vi "Prebuild Action VI.vi"(6 "Top Level/Always Included VIs":path[](array[path]), 7 "Main Destination Path":path, 9 "Target Name":string, 10 "Build Specification Name":string, 11 "Project Path":path) -> (0 "error out":errorcluster)   [LabVIEW 2018]
uses:
  <vilib>/AppBuilder/AB_API_Simple/Build Specification Version.ctl
  <vilib>/AppBuilder/AB_API_Simple/Get Build Specification Version (project reference).vi
  <vilib>/AppBuilder/AB_API_Simple/Set Build Specification Version (project reference).vi
  <vilib>/AppBuilder/AB_API_Simple/NI_App_Builder_API.lvlib
  <vilib>/Utility/config.llb/NI_LVConfig.lvlib
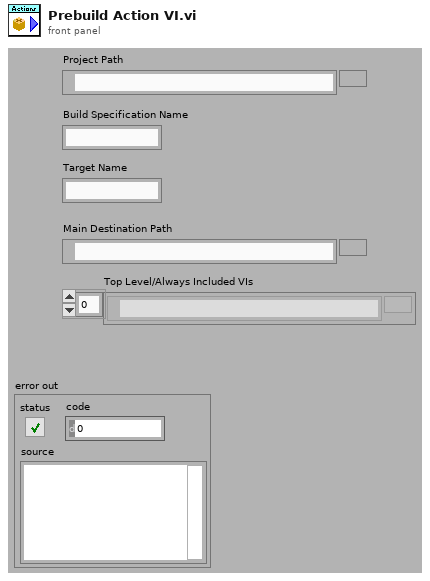
[diagram p1: front panel]
types:
  T1 = typedef "NI_App_Builder_API.lvlib/Build Specification Version.ctl" = cluster{"Major":u16, "Minor":u16, "Fix":u16, "Build":u16}
  T2 = cluster{"Major":bool, "Minor":bool, "Fix":bool, "Build":bool}
  T3 = typedef "NI_LVConfig.lvlib/Config Data RefNum.ctl" = refnum<k1>
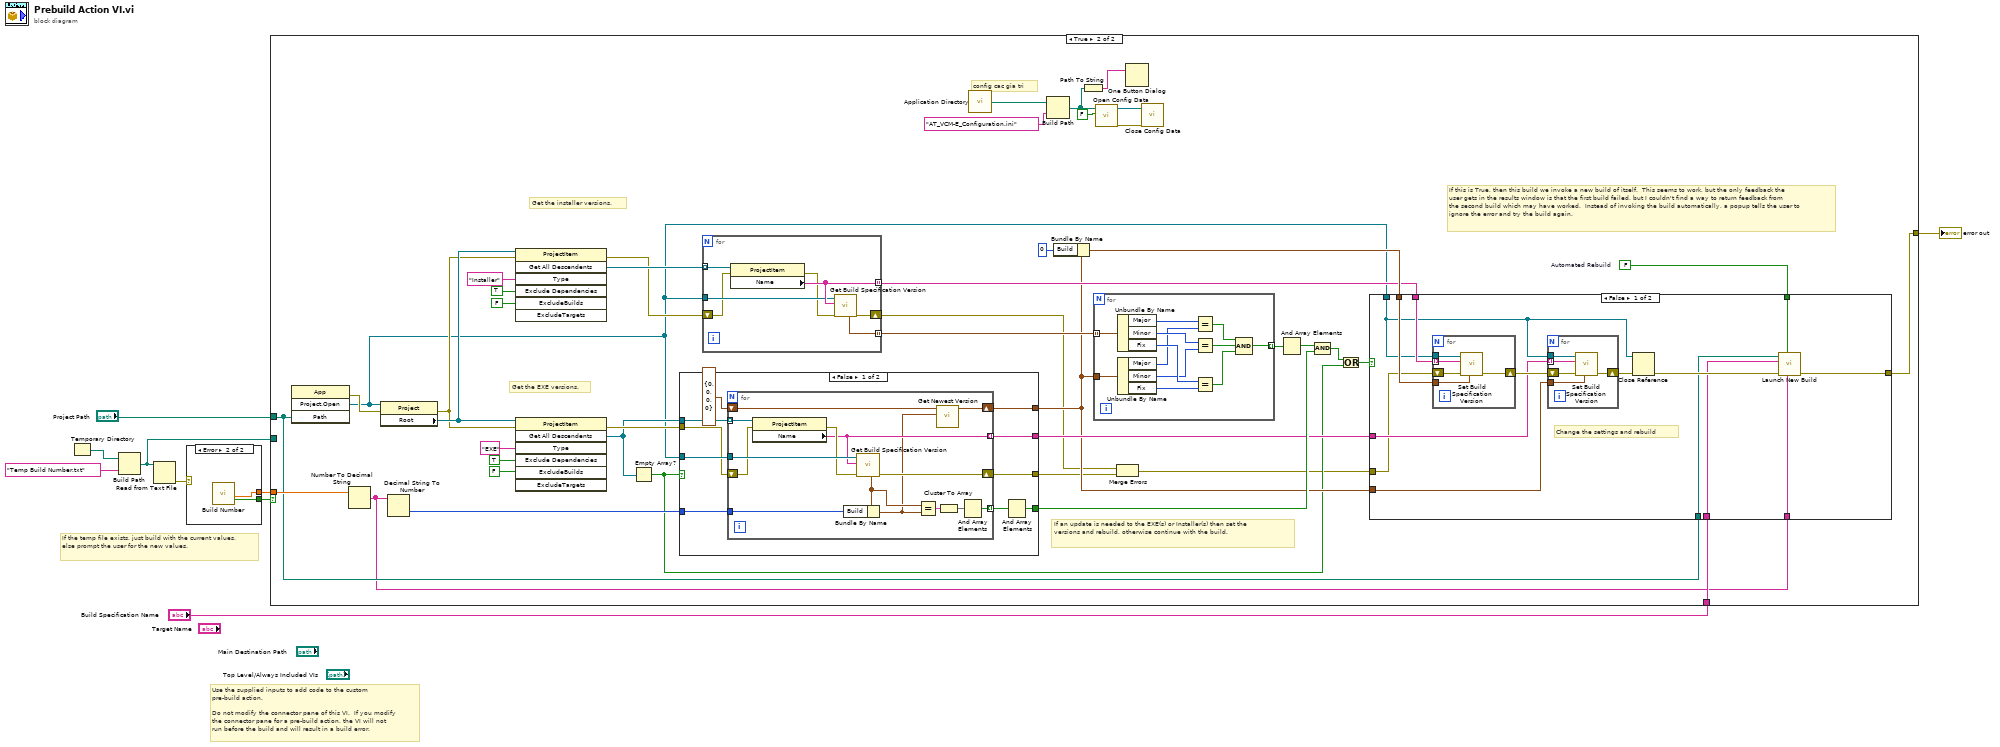
[diagram p0: block diagram]
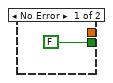
[diagram p2: hidden frame]
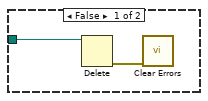
[diagram p3: hidden frame]
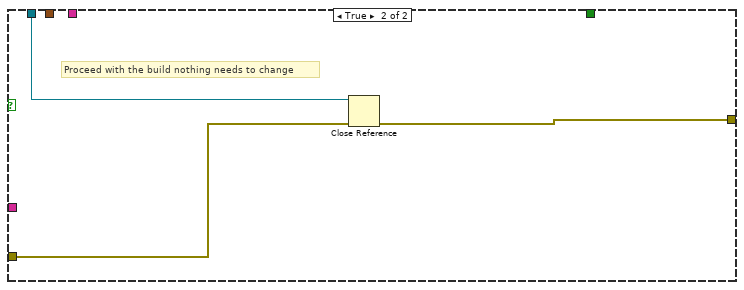
[diagram p5: hidden frame]
diagram:
  # "If the temp file exists, just build with the current values, else prompt the user for the new values."
  # "Use the supplied inputs to add code to the custom pre-build action.\n\nDo not modify the connector pane of this VI.  If you modify the connector pane for a pre-build action, the VI will not run before the build and will result in a build error."
  n1 = Temporary Directory() -> (w4:path)
  n2 = Build Path(base path=w4, name or relative path="Temp Build Number.txt") -> (appended path=w1:path)
  n3 = Read from Text File(file (use dialog)=w1) -> (error out=w2:errorcluster)  [unwired: 3 in, 3 out]
  n4 = case shown="Error" w2 {
    tunnel: [FALSE ("OK") w12] -> w7
    tunnel: [_ w11] -> w6
    frame No Error {
    }
    frame Error {
      n5 = call "Build Number"() -> ("Build Number"=w11:dbl, "OK"=w12:bool)  [unwired: 17 in, 1 out]
    }
  }
  n6 = case shown="True" w7 {
    tunnel: "Project Path" -> [_ w25]
    tunnel: [_ w24] -> w8
    tunnel: w6 -> [_ w49]
    tunnel: "Build Specification Name" -> [_ w27]
    tunnel: w1 -> [w14 _]
    frame False {
      n7 = Delete(path (use dialog)=w14) -> (error out=w13:errorcluster)  [unwired: 4 in, 2 out]
      n8 = call <vilib>:"Clear Errors.vi"("error in (no error)"=w13) -> ()  [unwired: 5 in, 2 out]
    }
    frame True {
      w23 = FALSE  # Automated Rebuild
      # "config cac gia tri"
      # "If an update is needed to the EXE(s) or Installer(s) then set the versions and rebuild, otherwise continue with the build."
      # "Get the EXE versions."
      # "Get the installer versions."
      # "If this is True, then this build we invoke a new build of itself.  This seems to work, but the only feedback the user gets in the results window is that the first build failed, but I couldn't find a way to return feedback from the second build which may have worked.  Instead of invoking the build automatically, a popup tells the user to ignore the error and try the build again."
      n9 = invoke class="App" method="Project.Open"("Path"=w25) -> (error out=w33:errorcluster, "Project:Open"=w26:refnum<vi>)  [unwired: 3 in, 2 out]
      n10 = Number To Decimal String(number=w49) -> (decimal integer string=w22:string)  [unwired: 1 in]
      n11 = property class="Project"(reference=w26, error in=w33) -> (error out=w35:errorcluster, "Root"=w50:refnum<vi>)  [unwired: 1 out]
      n12 = Decimal String To Number(string=w22) -> (number=w48:i32)  [unwired: 2 in, 1 out]
      n13 = invoke class="ProjectItem" method="Get All Descendents"(reference=w50, error in=w35, "Type"="Installer", "Exclude Dependencies"=TRUE ("ExcludeDependencies"), "ExcludeBuilds"=FALSE) -> (error out=w34:errorcluster, "All Descendents"=w51:refnum<vi>[])  [unwired: 2 in, 5 out]
      n14 = invoke class="ProjectItem" method="Get All Descendents"(reference=w50, error in=w35, "Type"="EXE", "Exclude Dependencies"=TRUE ("ExcludeDependencies"), "ExcludeBuilds"=FALSE) -> (error out=w43:errorcluster, "All Descendents"=w42:refnum<vi>[])  [unwired: 2 in, 5 out]
      n15 = Empty Array?(array=w42) -> (empty?=w31:bool)
      n16 = case shown="False" w31 {
        tunnel: w42 -> [w61 _]
        tunnel: w48 -> [w65 _]
        tunnel: w26 -> [w67 _]
        tunnel: [w60 _] -> w44
        tunnel: w43 -> [w66 w82]
        tunnel: [w63 w82] -> w30
        tunnel: [w62 _] -> w37
        tunnel: [w59 _] -> w36
        frame False {
          n17 = for {
            tunnel: w67 -> [w81]
            tunnel: w65 -> [w77]
            tunnel: [w75] -> w64 mode=indexing
            tunnel: [w73] -> w62 mode=indexing
            shift-right: [w74] -> w63
            shift-left: w66 -> [w79]
            tunnel: w61 -> [w72] mode=indexing
            shift-right: [w70] -> w59
            shift-left: T1 {"Major"=0, "Minor"=0, "Fix"=0, "Build"=0} ("Newest Version Out") -> [w69]
            n18 = property class="ProjectItem"(reference=w72, error in=w79) -> (error out=w78:errorcluster, "Name"=w73:string)  [unwired: 1 out]
            n19 = call-poly <vilib>:"Get Build Specification Version.vi"("error in (no error)"=w78, "Name of build specification"=w73, "Project reference"=w81) -> ("error out"=w74:errorcluster, "Build Specification Version"=w71:T1)  [unwired: 6 in, 1 out]
            n20 = Bundle By Name(cluster=w71, "Build"=w77) -> (w68:T1)
            n21 = Equal?(x=w71, y=w68) -> (x = y?=w80:T2)
            n22 = call "Get Newest Version.vi"("Version"=w68, "Newest Version In"=w69) -> ("Newest Version Out"=w70:T1)  [unwired: 9 in]
            n23 = Cluster To Array(cluster=w80) -> (array=w76:bool[])
            n24 = And Array Elements(Boolean array=w76) -> (logical AND=w75:bool)
          }
          n25 = And Array Elements(Boolean array=w64) -> (logical AND=w60:bool)
        }
        frame True {
        }
      }
      n26 = for {
        tunnel: w51 -> [w125] mode=indexing
        tunnel: [w128] -> w38 mode=indexing
        tunnel: w26 -> [w127]
        tunnel: [w126] -> w47 mode=indexing
        shift-right: [w123] -> w29
        shift-left: w34 -> [w122]
        n27 = property class="ProjectItem"(reference=w125, error in=w122) -> (error out=w124:errorcluster, "Name"=w128:string)  [unwired: 1 out]
        n28 = call-poly <vilib>:"Get Build Specification Version.vi"("error in (no error)"=w124, "Name of build specification"=w128, "Project reference"=w127) -> ("error out"=w123:errorcluster, "Build Specification Version"=w126:T1)  [unwired: 6 in, 1 out]
      }
      n29 = call <vilib>:"Application Directory.vi"() -> ("Application Directory"=w20:path)
      n30 = Build Path(base path=w20, name or relative path="AT_VCM-E_Configuration.ini") -> (appended path=w16:path)
      n31 = Bundle By Name(cluster=w36, "Build"=u16 0) -> (w39:T1)
      n32 = Path To String(path=w16) -> (string=w15:string)
      n33 = for {
        tunnel: w47 -> [w121] mode=indexing
        tunnel: w36 -> [w120]
        tunnel: [w110] -> w46 mode=indexing
        n34 = Unbundle By Name(w121) -> ("Major"=w119:u16, "Minor"=w118:u16, "Fix"=w117:u16)
        n35 = Unbundle By Name(w120) -> ("Major"=w114:u16, "Minor"=w115:u16, "Fix"=w116:u16)
        n36 = Equal?(x=w119, y=w114) -> (x = y?=w113:bool)
        n37 = Equal?(x=w118, y=w115) -> (x = y?=w112:bool)
        n38 = Equal?(x=w117, y=w116) -> (x = y?=w111:bool)
        n39 = Compound Arithmetic op=AND(w113, w112, w111) -> (w110:bool)
      }
      n40 = call <vilib>:"Open Config Data.vi"("create file if necessary (T)"=FALSE, "configuration file path"=w16) -> ("error out"=w17:errorcluster, "refnum"=w18:T3)  [unwired: 1 in, 7 out]
      n41 = Merge Errors(w29, w30) -> (w28:errorcluster)
      n42 = One Button Dialog(message=w15) -> ()  [unwired: 1 in, 1 out]
      n43 = call <vilib>:"Close Config Data.vi"("error in (no error)"=w17, "refnum"=w18) -> ()  [unwired: 8 in, 2 out]
      n44 = And Array Elements(Boolean array=w46) -> (logical AND=w45:bool)
      n45 = Compound Arithmetic op=AND(w45, w44) -> (w41:bool)
      n46 = Or(x=w41, y=w31) -> (x .or. y?=w32:bool)
      n47 = case shown="False" w32 {
        tunnel: w26 -> [w88 w107]
        tunnel: w39 -> [w96 _]
        tunnel: w38 -> [w95 _]
        tunnel: w36 -> [w93 _]
        tunnel: w37 -> [w92 _]
        tunnel: w28 -> [w91 w109]
        tunnel: [w84 w108] -> w24
        tunnel: w27 -> [w86 _]
        tunnel: w25 -> [w87 _]
        tunnel: w23 -> [w85 _]
        tunnel: w22 -> [w83 _]
        frame False {
          # "Change the settings and rebuild"
          n48 = for {
            tunnel: w88 -> [w106]
            tunnel: w96 -> [w105]
            tunnel: w95 -> [w104] mode=indexing
            shift-right: [w103] -> w94
            shift-left: w91 -> [w102]
            n49 = call-poly <vilib>:"Set Build Specification Version.vi"("Build Specification Version"=w105, "error in (no error)"=w102, "Name of build specification"=w104, "Project reference"=w106) -> ("error out"=w103:errorcluster)  [unwired: 6 in, 1 out]
          }
          n50 = for {
            tunnel: w88 -> [w101]
            tunnel: w93 -> [w100]
            tunnel: w92 -> [w99] mode=indexing
            shift-right: [w98] -> w90
            shift-left: w94 -> [w97]
            n51 = call-poly <vilib>:"Set Build Specification Version.vi"("Build Specification Version"=w100, "error in (no error)"=w97, "Name of build specification"=w99, "Project reference"=w101) -> ("error out"=w98:errorcluster)  [unwired: 6 in, 1 out]
          }
          n52 = Close Reference(reference=w88, error in (no error)=w90) -> (error out=w89:errorcluster)
          n53 = call "Launch New Build.vi"("Build Number"=w83, "Automated Rebuild"=w85, "error in (no error)"=w89, "Name of build specification (if empty: build all)"=w86, "Path to project"=w87) -> ("error out"=w84:errorcluster)  [unwired: 6 in]
        }
        frame True {
          # "Proceed with the build nothing needs to change"
          n54 = Close Reference(reference=w107, error in (no error)=w109) -> (error out=w108:errorcluster)
        }
      }
    }
  }
  "error out" <- w8
